vi "Begin.vi"(8 "error in (no error)":errorcluster, 11 "Vision in":refnum<class "Vision.lvclass">) -> (0 "error out":errorcluster, 3 "Vision out":refnum<class "Vision.lvclass">)   [LabVIEW 2018, in "Vision.lvlib" / "Vision.lvclass"]
doc: "This Vi sets camera mode in the limelight."
uses:
  Vision.lvclass
  <vilib>/Rock Robotics/Network Tables/NT Write Number.vi
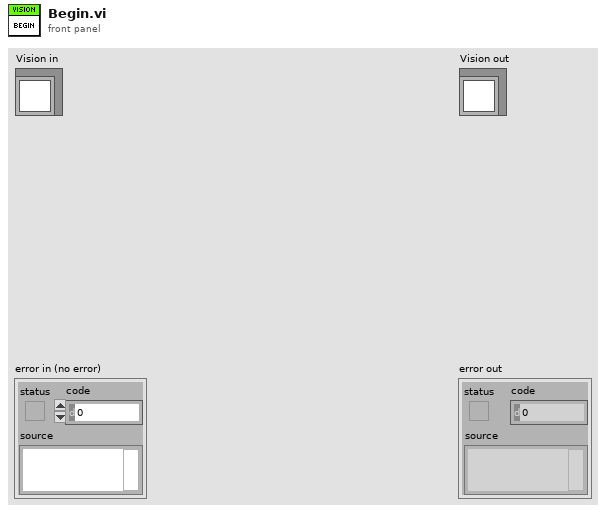
[diagram p1: front panel]
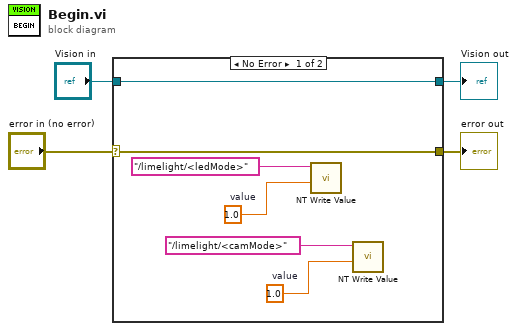
[diagram p0: block diagram]
diagram:
  n1 = case shown="No Error" "error in (no error)" {
    selector: "error in (no error)" -> [w10 w12]
    tunnel: [w10 w12] -> w3
    tunnel: [w9 w11] -> w1
    tunnel: "Vision in" -> [w9 w11]
    frame No Error {
      w6 = 1.0  # value
      w8 = 1.0  # value
      n2 = call-poly <vilib>:"NT Write Value.vi"("Numeric"=w6, "Name"="/limelight/<ledMode>") -> ()  [unwired: 9 in, 1 out]
      n3 = call-poly <vilib>:"NT Write Value.vi"("Numeric"=w8, "Name"="/limelight/<camMode>") -> ()  [unwired: 9 in, 1 out]
    }
    frame Error {
    }
  }
  "error out" <- w3
  "Vision out" <- w1
